vi "CN740_MODBUS_ASCII_sub_vi.vi"(6 "stop":T1, 8 "VISA PID":refnum<visa-resource-name>="COM6", 9 "DC Pulse (ON/OFF)":bool, 10 "Switch Mode":bool, 11 "SV":dbl=100.0 min=0.0 max=300.0 step=0.1 format="%.1f") -> ()   [LabVIEW 2023]
uses:
  <vilib>/Instr/_visa.llb/VISA Configure Serial Port (Instr).vi
  <extravilib>/ChannelInstances/Tag-bool.lvlib
  Control 1.ctl
panel:
  in  "Hysteresis":dbl=100.0 min=0.0 max=300.0 step=0.1 format="%.1f"
  out "Mode ON/OFF":bool
  out "Mode PID":bool
  out "PV":dbl format="%.1f"
  # "Real value"
  # "Target value"
  # "Only for on off"
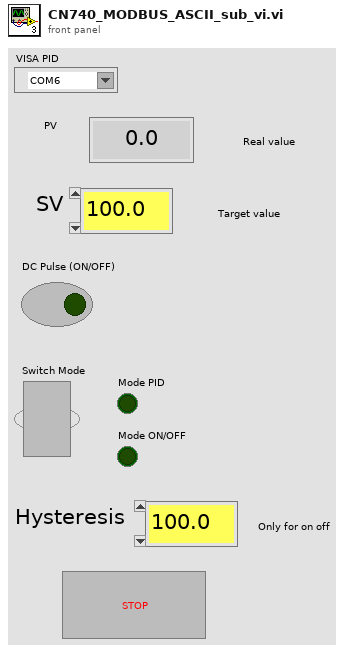
[diagram p1: front panel]
types:
  T1 = typedef "Control 1.ctl" = bool
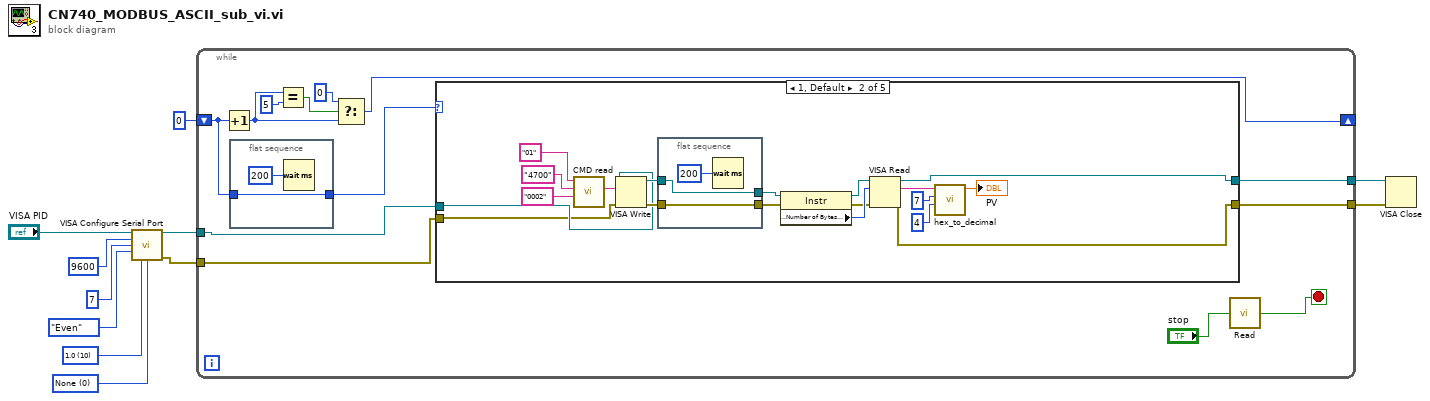
[diagram p0: block diagram]
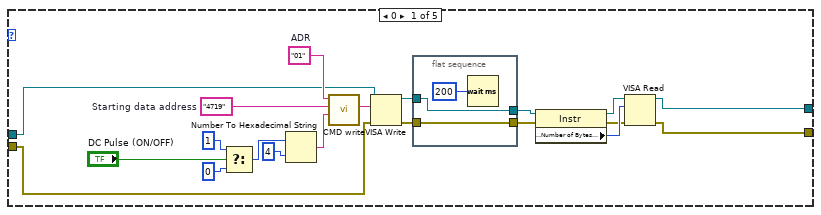
[diagram p2: hidden frame]
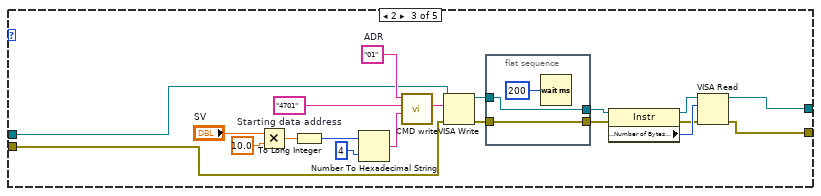
[diagram p3: hidden frame]
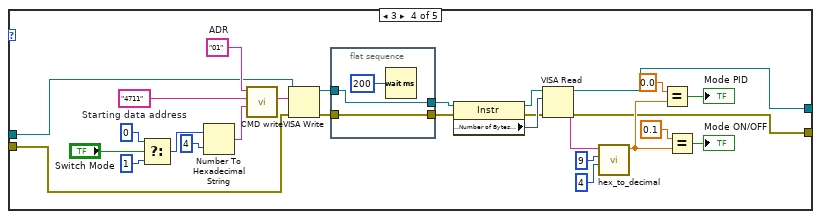
[diagram p4: hidden frame]
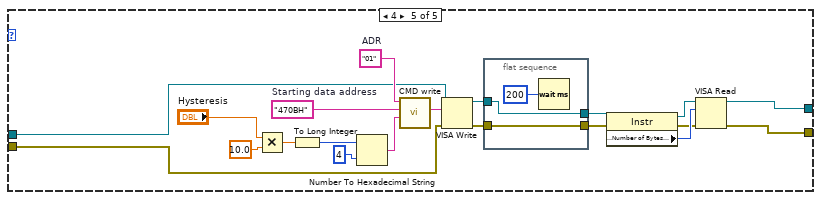
[diagram p5: hidden frame]
diagram:
  w6 = u16 0 items=["None"=0, "XON/XOFF"=1, "RTS/CTS"=2, "DTR/DSR"=4] ("flow control (0:none)")
  w7 = u16 10 items=["1.0"=10, "1.5"=15, "2.0"=20] ("stop bits (10: 1 bit)")
  n1 = call-poly "VISA Configure Serial Port"("VISA resource name"="VISA PID", "baud rate (9600)"=u32 9600, "data bits (8)"=u16 7, "parity (0:none)"=enum16{"None", "Odd", "Even", "Mark", "Space"}."Even", "stop bits (10: 1 bit)"=w7, "flow control (0:none)"=w6) -> ("VISA resource name out"=w5:refnum<visa-resource-name>, "error out"=w4:errorcluster)  [unwired: 2 in, 6 out]
  n2 = while {
    tunnel: w5 -> [w19]
    tunnel: w4 -> [w18]
    shift-right: [w16] -> _
    shift-left: 0 -> [w17]
    tunnel: [w15] -> w2
    tunnel: [w14] -> w1
    stop <- w13 stop-if-true
    n3 = Increment(x=w17) -> (x+1=w22:i32)
    n4 = flat-sequence {
      tunnel: w17 -> [w25]
      tunnel: [w25] -> w20
      frame #0 {
        n5 = Wait (ms)(milliseconds to wait=u32 200 ("attente (ms)")) -> ()  [unwired: 1 out]
      }
    }
    n6 = Equal?(x=w22, y=5) -> (x = y?=w23:bool)
    n7 = Select(t=0, s=w23, f=w22) -> (s? t:f=w16:i32)
    n8 = case shown="1, Default" w20 {
      tunnel: w19 -> [w30 w53 w75 w107 w130]
      tunnel: w18 -> [w29 w52 w74 w106 w129]
      tunnel: [w28 w51 w73 w96 w128] -> w15
      tunnel: [w27 w50 w72 w95 w127] -> w14
      frame 0 {
        w39 = "01"  # ADR
        w38 = "4719"  # Starting data address
        n9 = Select(t=1, s="DC Pulse (ON/OFF)", f=0) -> (s? t:f=w33:i32)
        n10 = Number To Hexadecimal String(1:i16 4 ("largeur (-)"), 2:w33) -> (0:w31:string)
        n11 = call "CMD write.vi"("Data Content"=w31, "Starting data address"=w38, "ADR"=w39) -> ("Chaîne en sortie"=w37:string)  [unwired: 6 in]
        n12 = VISA Write(VISA resource name=w30, write buffer=w37, error in (no error)=w29) -> (VISA resource name out=w43:refnum<visa-resource-name>, error out=w40:errorcluster)  [unwired: 1 out]
        n13 = flat-sequence {
          tunnel: w43 -> [w48]
          tunnel: [w48] -> w42
          tunnel: [w47] -> w41
          tunnel: w40 -> [w47]
          frame #0 {
            n14 = Wait (ms)(milliseconds to wait=u32 200 ("attente (ms)")) -> ()  [unwired: 1 out]
          }
        }
        n15 = property class="Instr"(reference=w42, error in=w41) -> (reference out=w46:refnum<visa-resource-name>, error out=w44:errorcluster, "Serial Settings:Number of Bytes at Serial Port"=w45:u32)
        n16 = VISA Read(VISA resource name=w46, byte count=w45, error in (no error)=w44) -> (VISA resource name out=w28:refnum<visa-resource-name>, error out=w27:errorcluster)  [unwired: 2 out]
      }
      frame 1, Default {
        n17 = call "CMD read.vi"("Data Content"="0002", "Starting data address"="4700", "ADR"="01") -> ("Chaîne en sortie"=w55:string)  [unwired: 6 in]
        n18 = VISA Write(VISA resource name=w53, write buffer=w55, error in (no error)=w52) -> (VISA resource name out=w65:refnum<visa-resource-name>, error out=w62:errorcluster)  [unwired: 1 out]
        n19 = flat-sequence {
          tunnel: w65 -> [w70]
          tunnel: [w70] -> w64
          tunnel: [w69] -> w63
          tunnel: w62 -> [w69]
          frame #0 {
            n20 = Wait (ms)(milliseconds to wait=u32 200 ("attente (ms)")) -> ()  [unwired: 1 out]
          }
        }
        n21 = property class="Instr"(reference=w64, error in=w63) -> (reference out=w68:refnum<visa-resource-name>, error out=w66:errorcluster, "Serial Settings:Number of Bytes at Serial Port"=w67:u32)
        n22 = VISA Read(VISA resource name=w68, byte count=w67, error in (no error)=w66) -> (VISA resource name out=w51:refnum<visa-resource-name>, read buffer=w54:string, error out=w50:errorcluster)  [unwired: 1 out]
        n23 = call "hex_to_decimal.vi"("length (rest)"=4, "offset (0)"=7, "read buffer"=w54) -> ("Numeric"=→"PV":dbl)  [unwired: 8 in]
      }
      frame 2 {
        w79 = "01"  # ADR
        w77 = "4701"  # Starting data address
        n24 = Multiply(x="SV", y=10.0) -> (x*y=w87:dbl)
        n25 = To Long Integer(number=w87) -> (32bit integer=w91:i32)
        n26 = Number To Hexadecimal String(1:i16 4 ("largeur (-)"), 2:w91) -> (0:w78:string)
        n27 = call "CMD write.vi"("Data Content"=w78, "Starting data address"=w77, "ADR"=w79) -> ("Chaîne en sortie"=w76:string)  [unwired: 6 in]
        n28 = VISA Write(VISA resource name=w75, write buffer=w76, error in (no error)=w74) -> (VISA resource name out=w83:refnum<visa-resource-name>, error out=w80:errorcluster)  [unwired: 1 out]
        n29 = flat-sequence {
          tunnel: w83 -> [w93]
          tunnel: [w93] -> w82
          tunnel: [w92] -> w81
          tunnel: w80 -> [w92]
          frame #0 {
            n30 = Wait (ms)(milliseconds to wait=u32 200 ("attente (ms)")) -> ()  [unwired: 1 out]
          }
        }
        n31 = property class="Instr"(reference=w82, error in=w81) -> (reference out=w86:refnum<visa-resource-name>, error out=w84:errorcluster, "Serial Settings:Number of Bytes at Serial Port"=w85:u32)
        n32 = VISA Read(VISA resource name=w86, byte count=w85, error in (no error)=w84) -> (VISA resource name out=w73:refnum<visa-resource-name>, error out=w72:errorcluster)  [unwired: 2 out]
      }
      frame 3 {
        w115 = "01"  # ADR
        w114 = "4711"  # Starting data address
        n33 = Select(t=0, s="Switch Mode", f=1) -> (s? t:f=w110:i32)
        n34 = Number To Hexadecimal String(1:i16 4 ("largeur (-)"), 2:w110) -> (0:w108:string)
        n35 = call "CMD write.vi"("Data Content"=w108, "Starting data address"=w114, "ADR"=w115) -> ("Chaîne en sortie"=w113:string)  [unwired: 6 in]
        n36 = VISA Write(VISA resource name=w107, write buffer=w113, error in (no error)=w106) -> (VISA resource name out=w119:refnum<visa-resource-name>, error out=w116:errorcluster)  [unwired: 1 out]
        n37 = flat-sequence {
          tunnel: w119 -> [w124]
          tunnel: [w124] -> w118
          tunnel: [w123] -> w117
          tunnel: w116 -> [w123]
          frame #0 {
            n38 = Wait (ms)(milliseconds to wait=u32 200 ("attente (ms)")) -> ()  [unwired: 1 out]
          }
        }
        n39 = property class="Instr"(reference=w118, error in=w117) -> (reference out=w122:refnum<visa-resource-name>, error out=w120:errorcluster, "Serial Settings:Number of Bytes at Serial Port"=w121:u32)
        n40 = VISA Read(VISA resource name=w122, byte count=w121, error in (no error)=w120) -> (VISA resource name out=w96:refnum<visa-resource-name>, read buffer=w103:string, error out=w95:errorcluster)  [unwired: 1 out]
        n41 = call "hex_to_decimal.vi"("length (rest)"=4, "offset (0)"=9, "read buffer"=w103) -> ("Numeric"=w101:dbl)  [unwired: 8 in]
        n42 = Equal?(x=0.0, y=w101) -> (x = y?=→"Mode PID":bool)
        n43 = Equal?(x=0.1, y=w101) -> (x = y?=→"Mode ON/OFF":bool)
      }
      frame 4 {
        w134 = "01"  # ADR
        w132 = "470BH"  # Starting data address
        n44 = Multiply(x="Hysteresis", y=10.0) -> (x*y=w142:dbl)
        n45 = To Long Integer(number=w142) -> (32bit integer=w145:i32)
        n46 = Number To Hexadecimal String(1:i16 4 ("largeur (-)"), 2:w145) -> (0:w133:string)
        n47 = call "CMD write.vi"("Data Content"=w133, "Starting data address"=w132, "ADR"=w134) -> ("Chaîne en sortie"=w131:string)  [unwired: 6 in]
        n48 = VISA Write(VISA resource name=w130, write buffer=w131, error in (no error)=w129) -> (VISA resource name out=w138:refnum<visa-resource-name>, error out=w135:errorcluster)  [unwired: 1 out]
        n49 = flat-sequence {
          tunnel: w138 -> [w147]
          tunnel: [w147] -> w137
          tunnel: [w146] -> w136
          tunnel: w135 -> [w146]
          frame #0 {
            n50 = Wait (ms)(milliseconds to wait=u32 200 ("attente (ms)")) -> ()  [unwired: 1 out]
          }
        }
        n51 = property class="Instr"(reference=w137, error in=w136) -> (reference out=w141:refnum<visa-resource-name>, error out=w139:errorcluster, "Serial Settings:Number of Bytes at Serial Port"=w140:u32)
        n52 = VISA Read(VISA resource name=w141, byte count=w140, error in (no error)=w139) -> (VISA resource name out=w128:refnum<visa-resource-name>, error out=w127:errorcluster)  [unwired: 2 out]
      }
    }
    n53 = call <extravilib>:"Read.vi"("channel"="stop") -> ("element"=w13:bool)  [unwired: 1 in, 1 out]
  }
  n54 = VISA Close(VISA resource name=w2, error in (no error)=w1) -> ()  [unwired: 1 out]
